vi "Generate Test Report.vi"(7 "Print Report?":bool=TRUE, 8 "error in":errorcluster, 11 "Sequence Context In":T1) -> (0 "error out":errorcluster, 3 "Sequence Context Out":T1)   [LabVIEW 2010]
uses:
  <vilib>/addons/TestStand/_TSLegacy.llb/LabVIEW Test - Sequence Context.ctl
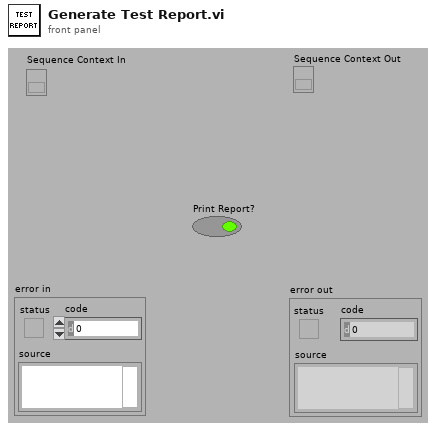
[diagram p1: front panel]
types:
  T1 = typedef "LabVIEW Test - Sequence Context.ctl" = refnum<k7>
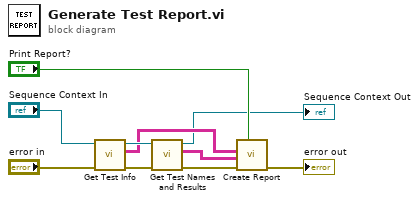
[diagram p0: block diagram]
diagram:
  n1 = call "Get Test Info.vi"("error in (no error)"="error in", "Sequence Context In"="Sequence Context In") -> ("error out"=w10:errorcluster, "Test Results"=w3:string[][], "Sequence Context out"=w9:T1)  [unwired: 6 in]
  n2 = call "Get Test Names and Results.vi"("error in (no error)"=w10, "Sequence Context In"=w9) -> ("error out"=w5:errorcluster, "Test Results"=w4:string[][], "Sequence Context Out"=→"Sequence Context Out":T1)  [unwired: 7 in]
  n3 = call "Create Report.vi"("Print Report?"="Print Report?", "error in"=w5, "Test Results"=w4, "Test Info"=w3) -> ("error out"=→"error out":errorcluster)  [unwired: 7 in]
